vi "CRYStep Default.vi"(11 "Category Name":string="stimulus.txt") -> (0 "status":bool, 3 "Flatten Step":string)   [LabVIEW 2013]
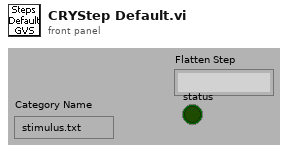
[diagram p1: front panel]
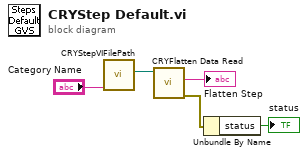
[diagram p0: block diagram]
diagram:
  n1 = call "CRYStepVIFilePath.vi"("Category Name"="Category Name") -> ("Default StepFilePath"=w1:path)  [unwired: 1 in, 8 out]
  n2 = call "CRYFlatten Data Read.vi"("Path In"=w1) -> ("error out"=w3:errorcluster, "Flatten Data Out"=→"Flatten Step":string)  [unwired: 6 in, 1 out]
  n3 = Unbundle By Name(w3) -> ("status"=→"status":bool)
